vi "Test Notifiers.vi"() -> ()   [LabVIEW 2019, in "Inst.Transport.lvclass"]
uses:
  Inst.Transport.lvclass
  Inst.Transport.lvclass/Inst.Transport.ctl
panel:
  out "Numeric 1":i32
  out "Numeric 2":i32
  in  "stop":bool
  out "latest notification":bool
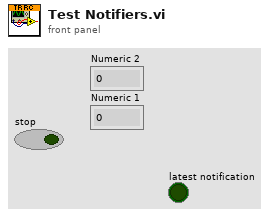
[diagram p1: front panel]
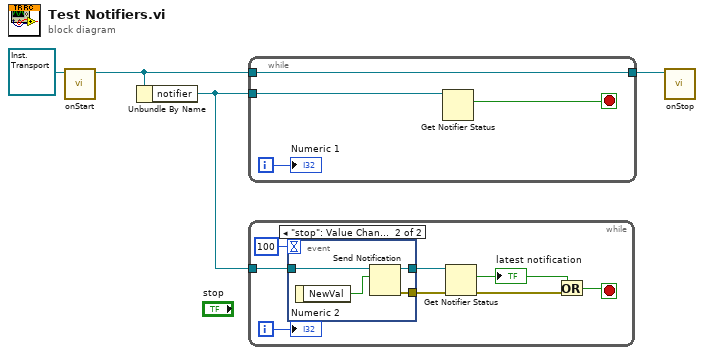
[diagram p0: block diagram]
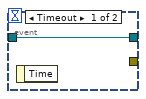
[diagram p2: hidden frame]
diagram:
  n1 = call-dynamic "onStart.vi"("Inst.Transport"=refnum<class "Inst.Transport.lvclass"> refnum) -> ("Inst.Transport out"=w1:refnum<class "Inst.Transport.lvclass">)  [unwired: 9 in, 1 out]
  n2 = Unbundle By Name(w1) -> ("notifier"=w3:refnum<notifier>)
  n3 = while {
    tunnel: w3 -> [w5]
    tunnel: [w8] -> w2
    tunnel: w1 -> [w8]
    i -> [w7]
    stop <- w6 stop-if-true
    n4 = Get Notifier Status(notifier=w5) -> (current notification=w6:bool)  [unwired: 1 in, 4 out]
    "Numeric 1" <- w7
  }
  n5 = while {
    tunnel: w3 -> [w16]
    i -> [w9]
    stop <- w12 stop-if-true
    n6 = event shown="[1] \"stop\": Value Change" {
      selector: _ -> [_ _]
      dyn-events: _ -> [_ _]
      timeout: 100 -> [_ _]
      tunnel: w16 -> [w17 w21]
      tunnel: [w17 w20] -> w15
      tunnel: [_ w19] -> w14
      event Timeout {
        n7 = event-data() -> ()  [unwired: 1 in, 1 out]
      }
      event "stop": Value Change {
        n8 = event-data() -> ("NewVal"=w18:bool)  [unwired: 1 in]
        n9 = Send Notification(notification=w18, notifier=w21) -> (notifier out=w20:refnum<notifier>, error out=w19:errorcluster)  [unwired: 1 in]
      }
    }
    n10 = Get Notifier Status(notifier=w15, error in (no error)=w14) -> (current notification=w11:bool, error out=w10:errorcluster)  [unwired: 3 out]
    "latest notification" <- w11
    n11 = Or(x=w11, y=w10) -> (x .or. y?=w12:bool)
    "Numeric 2" <- w9
  }
  n12 = call-dynamic "onStop.vi"("Inst.Transport"=w2) -> ()  [unwired: 9 in, 2 out]
